vi "UpdateBlockDataRamp.vi"(5 "BlockUpdate":bool) -> ()   [LabVIEW 2016]
uses:
  controls/Enum.ctl
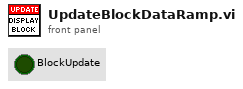
[diagram p1: front panel]
types:
  T1 = typedef "Enum.ctl" = enum16{"Init", "Read", "Write"}
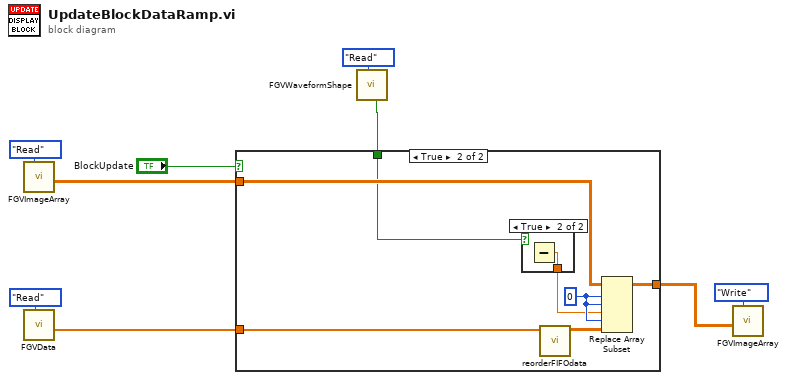
[diagram p0: block diagram]
diagram:
  n1 = call "FGVImageArray.vi"("Enum"=Enum."Read") -> ("imageArrayOut"=w5:sgl[][][][])  [unwired: 9 in, 1 out]
  n2 = call "FGVData.vi"("Enum"=Enum."Read") -> ("DataOut"=w1:dbl[])  [unwired: 9 in, 1 out]
  n3 = call "FGVWaveformShape.vi"("Enum"=Enum."Read") -> ("Framing up? (down: f)"=w7:bool)  [unwired: 6 in, 4 out]
  n4 = case shown="True" "BlockUpdate" {
    tunnel: w5 -> [w10 w16]
    tunnel: [w10 w15] -> w3
    tunnel: w1 -> [_ w14]
    tunnel: w7 -> [_ w13]
    frame False {
    }
    frame True {
      w17 = 0 ("disabled index (vol)")
      n5 = case shown="True" w13 {
        tunnel: [_ w18] -> w12
        frame False {
        }
        frame True {
          n6 = Subtract() -> (x-y=w18:dbl)  [unwired: 2 in]
        }
      }
      n7 = call "reorderFIFOdata.vi"("inputElements"=w14) -> ("outputElements"=w11:sgl[][][][])  [unwired: 10 in]
      n8 = Replace Array Subset(array=w16, new element=w11, index (dim 0)=w17, index (dim 1)=w17, index (dim 2)=w12, index (dim 3)=w17) -> (w15:sgl[][][][])
    }
  }
  n9 = call "FGVImageArray.vi"("Enum"=Enum."Write", "imageArrayIn"=w3) -> ()  [unwired: 8 in, 2 out]
